vi "003 Treu tres missatges pantalla.vi"   [LabVIEW 2019]
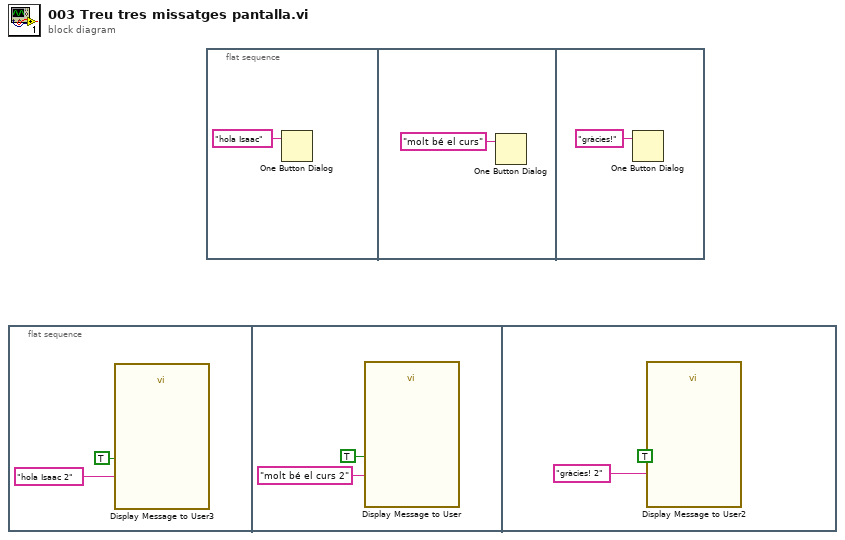
[diagram p0: block diagram]
diagram:
  n1 = flat-sequence {
    frame #0 {
      n2 = call "Display Message to User3"("Enable"=TRUE, "Message"="hola Isaac 2" ("message")) -> ()  [unwired: 8 in, 2 out]
    }
    frame #1 {
      n3 = call "Display Message to User"("Enable"=TRUE, "Message"="molt bé el curs 2" ("message")) -> ()  [unwired: 8 in, 2 out]
    }
    frame #2 {
      n4 = call "Display Message to User2"("Enable"=TRUE, "Message"="gràcies! 2" ("message")) -> ()  [unwired: 8 in, 2 out]
    }
  }
  n5 = flat-sequence {
    frame #0 {
      n6 = One Button Dialog(message="hola Isaac") -> ()  [unwired: 1 in, 1 out]
    }
    frame #1 {
      n7 = One Button Dialog(message="molt bé el curs") -> ()  [unwired: 1 in, 1 out]
    }
    frame #2 {
      n8 = One Button Dialog(message="gràcies!") -> ()  [unwired: 1 in, 1 out]
    }
  }
